vi "Update.vi"(8 "error in (no error)":errorcluster, 11 "Simple Actor in":refnum<class "Simple Actor.lvclass">) -> (0 "error out":errorcluster, 3 "Simple Actor out":refnum<class "Simple Actor.lvclass">)   [LabVIEW 2012, in "Simple Actor.lvclass"]
uses:
  Simple Actor.lvclass
  Simple Actor.lvclass/Simple Actor.ctl
  <vilib>/ptbypt/NI_PtbyPt.lvlib
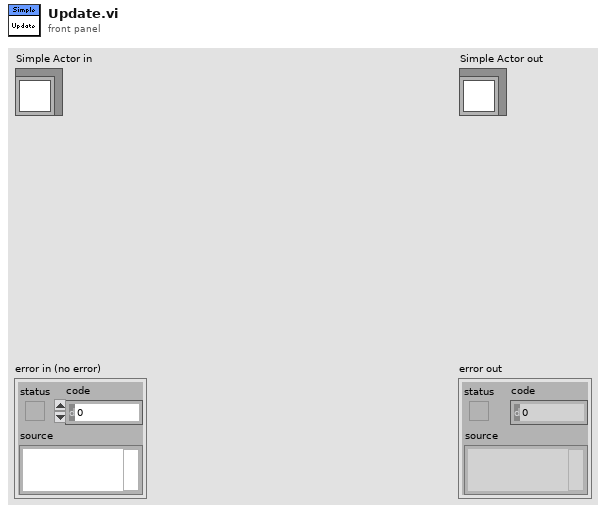
[diagram p1: front panel]
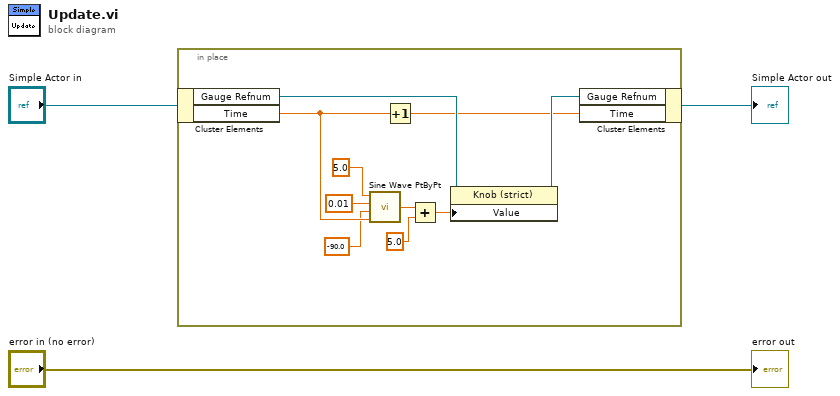
[diagram p0: block diagram]
diagram:
  n1 = in-place {
    n2 = in-place-cluster #1("Simple Actor in") -> ("Gauge Refnum"=w10:refnum<vi>, "Time"=w8:dbl)
    n3 = call <vilib>:"Sine Wave PtByPt.vi"("time"=w8, "phase"=-90.0, "frequency"=0.01, "amplitude"=5.0) -> ("sine wave"=w11:dbl)
    n4 = Increment(x=w8) -> (x+1=w7:dbl)
    n5 = Add(x=w11, y=5.0) -> (x+y=w6:dbl)
    n6 = property class="Knob (strict)"(reference=w10, "Value"=w6) -> (reference out=w9:refnum<vi>)  [unwired: 1 in, 1 out]
    n7 = in-place-cluster #1("Gauge Refnum"=w9, "Time"=w7) -> (→"Simple Actor out":refnum<class "Simple Actor.lvclass">)
  }
  "error out" <- "error in (no error)"
